vi "gentec-M-Link.Get Range.vi"(0 "VISA resource In":refnum<visa-resource-name>, 2 "Range Queries":T1="VER", 5 "error in (no error)":errorcluster) -> (11 "Data Read":string, 13 "Read Timeout":bool, 14 "VISA resource Out":refnum<visa-resource-name>, 16 "Range":T2 items=["1f", "3f", "10f", "30f", "100f", "300f", "1p", "3p", "10p", "30p", "100p", "300p", "1n", "3n", "10n", "30n", "100n", "300n", "1u", "3u", "10u", "30u", "100u", "300u", "1m", "3m", "10m", "30m", "100m", "300m", "1", "3", "10", "30", "100", "300", "1K", "3K", "10K", "30K", "100K", "300K", "1M", "3M", "10M", "30M", "100M", "300M"], 17 "Error":bool, 19 "error out":errorcluster)   [LabVIEW 2014, in "gentec-M-Link - Driver.lvlib"]
doc: "Data to write: rng, min, or max\n\nQueries the current, minimum or maximum instrument range for the head in use."
uses:
  gentec-M-Link - Driver.lvlib
  Type Defs/gentec-M-Link.Range.ctl
  Type Defs/gentec-M-Link.Range Queries.ctl
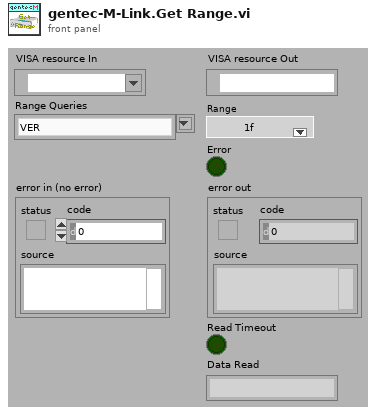
[diagram p1: front panel]
types:
  T1 = typedef "gentec-M-Link - Driver.lvlib/gentec-M-Link.Range Queries.ctl" = string
  T2 = typedef "gentec-M-Link - Driver.lvlib/gentec-M-Link.Range.ctl" = u16
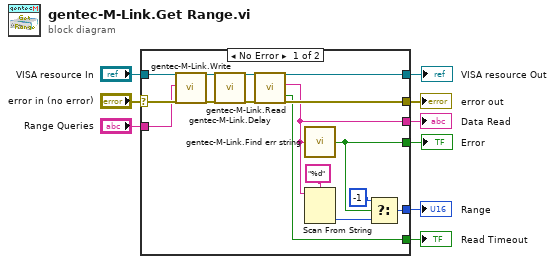
[diagram p0: block diagram]
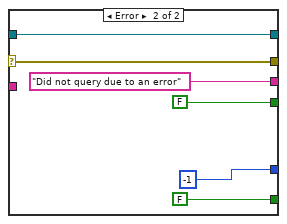
[diagram p2: hidden frame]
diagram:
  n1 = case shown="No Error" "error in (no error)" {
    selector: "error in (no error)" -> [w22 w31]
    tunnel: [w23 w31] -> w8
    tunnel: "VISA resource In" -> [w21 w30]
    tunnel: [w20 w30] -> w6
    tunnel: [w12 -1] -> w5
    tunnel: [w15 "Did not query due to an error" ("Data Read")] -> w4
    tunnel: [w16 FALSE ("Read Timeout")] -> w3
    tunnel: [w14 FALSE ("Found")] -> w2
    tunnel: "Range Queries" -> [w10 _]
    frame No Error {
      n2 = call "gentec-M-Link.Write.vi"("VISA resource (In)"=w21, "Data To Write"=w10, "error in (no error)"=w22) -> ("VISA resource (Out)"=w25:refnum<visa-resource-name>, "error out"=w24:errorcluster)  [unwired: 14 in, 1 out]
      n3 = call "gentec-M-Link.Delay.vi"("VISA resource In"=w25, "error in (no error)"=w24) -> ("VISA resource Out"=w19:refnum<visa-resource-name>, "error out"=w18:errorcluster)  [unwired: 16 in]
      n4 = call "gentec-M-Link.Read.vi"("VISA resource (In)"=w19, "error in (no error)"=w18) -> ("VISA resource (Out)"=w20:refnum<visa-resource-name>, "Data Read"=w15:string, "Read Timeout"=w16:bool, "error out"=w23:errorcluster)  [unwired: 13 in, 1 out]
      n5 = call "gentec-M-Link.Find err string.vi"("string"=w15) -> ("Found"=w14:bool)
      n6 = Scan From String(format string="%d", input string=w15) -> (output 1=w13:i32)  [unwired: 3 in, 3 out]
      n7 = Select(t=-1, s=w14, f=w13) -> (s? t:f=w12:i32)
    }
    frame Error {
    }
  }
  "error out" <- w8
  "VISA resource Out" <- w6
  "Range" <- w5
  "Data Read" <- w4
  "Read Timeout" <- w3
  "Error" <- w2
